vi "Starter Kit 2.0 Robot Receiver.vi"() -> ()   [LabVIEW 2010]
doc: "This VI runs on the Starter Kit RT target. Run this VI before running the host controller VI. You can build this VI into a startup application so that it runs on the robot whenever the RT target is powered on."
uses:
  <vilib>/Platform/TimedLoop/XDataNode/XDataNode.xnode
  <vilib>/Platform/TimedLoop/XDataNode/timing_clust.ctl
  <vilib>/Platform/TimedLoop/XDataNode/nitl_modes.ctl
  <vilib>/Platform/TimedLoop/XDataNode/wakeup.ctl
  Support VIs/Motor Velocity.ctl
  <vilib>/robotics/Starter Kit/2.0/9632 Host Interface/NI_Robotics_Starter Kit Host_9632_2.0.lvclass
  <vilib>/Platform/TimedLoop/XDataNode/XDNodeRunTimeDep.lvlib
  <vilib>/robotics/Starter Kit/Host Interface/NI_Robotics_Starter Kit Host.lvclass
  <vilib>/NI_Real-Time Target Support.lvlib
panel:
  out "connection":i32
  in  "stop":bool
  in  "port (12345)":u16=12345
  in  "ccw servo angle (rad)":dbl
  in  "right motor ccw vel sp":dbl
  in  "left motor ccw vel sp":dbl
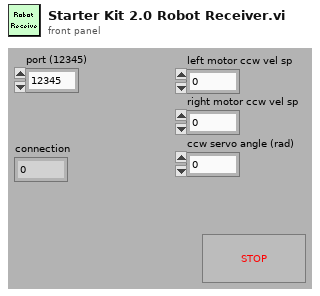
[diagram p1: front panel]
types:
  T1 = typedef "XDNodeRunTimeDep.lvlib/timing_clust.ctl" = cluster{"Expected End [f-1]":u64, "Actual End [f-1]":u64, "Finished Late? [f-1]":bool, "Expected End [i-1]":u64, "Actual End [i-1]":u64, "Finished Late? [i-1]":bool, "Expected Start [i]":u64, "Actual Start [i]":u64, "Expected Start [f]":u64, "Actual Start [f]":u64, "Source Name":string, "Structure Name":string, "Period":i64, "Deadline":i64, "Offset":i64, "Start":i64, "Priority":i32, "Timeout":i32, "Mode":T2, "Wakeup Reason":T3, "Error":errorcluster, "Source Type":string, "Secondary Source Type":string, "Global End Time":u64, "Global Start Time":u64, "Frame Duration":u64, "Iteration Duration":u64, "Assigned CPU":i32, "I/O Scan Engine Mode":u32}
  T2 = typedef "XDNodeRunTimeDep.lvlib/nitl_modes.ctl" = enum32{"No Change", "Process missed periods, maintain original phase", "Discard missed periods, maintain original phase", "Process missed periods, ignore original phase", "Discard missed periods, ignore original phase"}
  T3 = typedef "XDNodeRunTimeDep.lvlib/wakeup.ctl" = enum32{"Normal", "Aborted", "Asynchronous wakeup", "Timing source error", "Timed loop error", "Timeout"}
  T4 = typedef "Motor Velocity.ctl" = cluster{"left motor ccw vel":dbl, "right motor ccw vel":dbl}
  T5 = typedef "Starter Kit Message.ctl" = cluster{"message type":enum16{"Heartbeat", "Motor Vel SP", "Servo Angle", "Stop"}, "message data":variant}
  T6 = enum16{"Heartbeat", "Motor Vel SP", "Servo Angle", "Stop"}
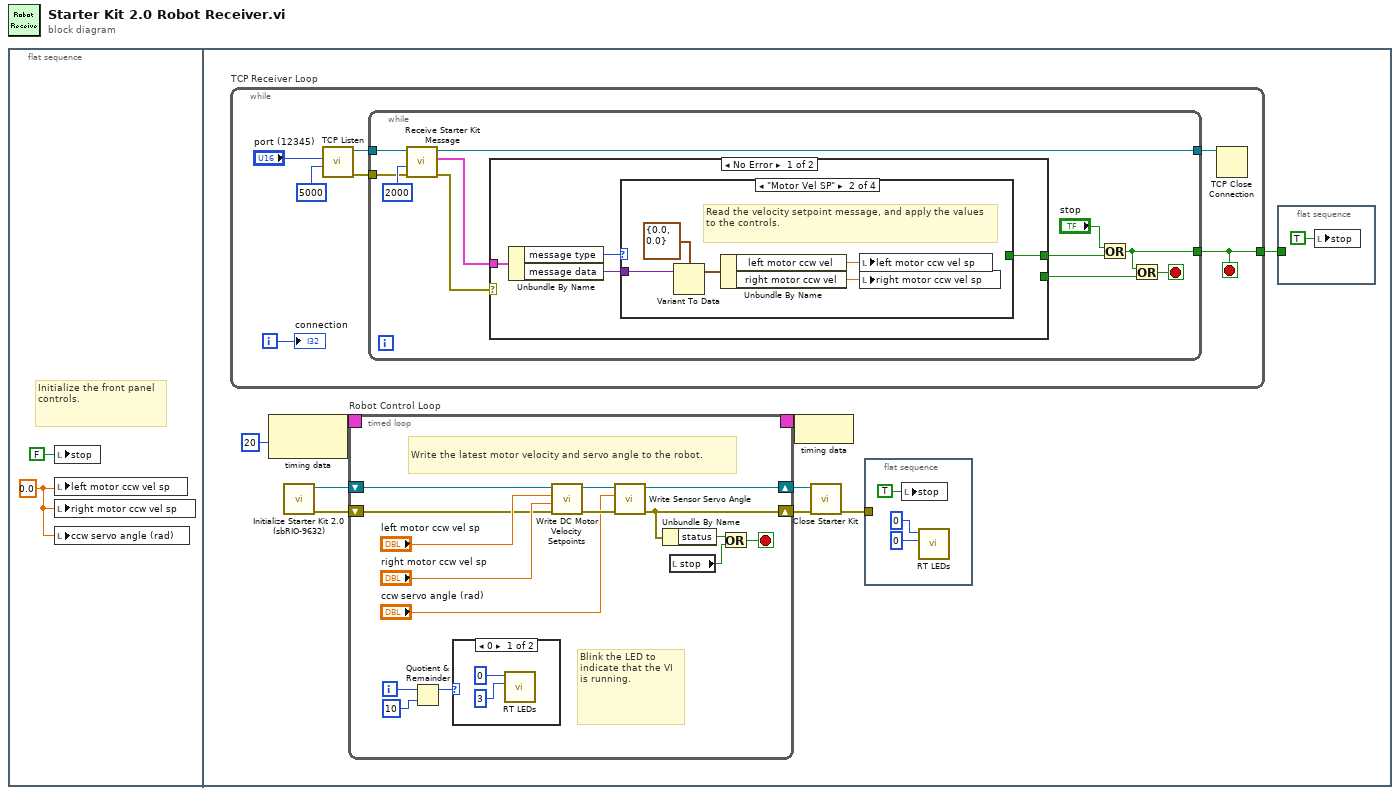
[diagram p0: block diagram]
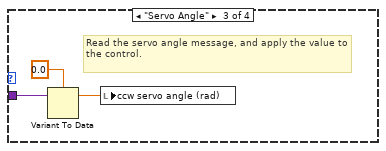
[diagram p4: hidden frame]
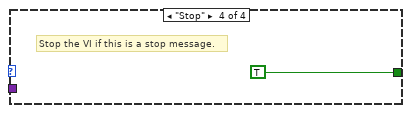
[diagram p5: hidden frame]
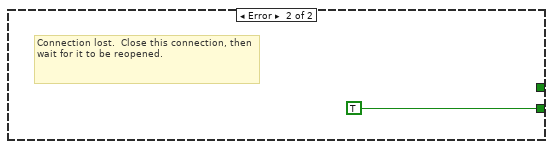
[diagram p6: hidden frame]
diagram:
  n1 = flat-sequence {
    frame #0 {
      w1 = 0.0 ("left motor ccw vel sp")
      # "Initialize the front panel controls."
      n2 = local write "stop"(FALSE ("stop")) -> ()
      n3 = local write "left motor ccw vel sp"(w1) -> ()
      n4 = local write "right motor ccw vel sp"(w1) -> ()
      n5 = local write "ccw servo angle (rad)"(w1) -> ()
    }
    frame #1 {
      n6 = while "TCP Receiver Loop" {
        tunnel: [w40] -> w11
        i -> [w39]
        stop <- w40 stop-if-true
        n7 = call <vilib>:"TCP Listen.vi"("timeout ms (wait forever: -1)"=5000, "port"="port (12345)") -> ("error out"=w41:errorcluster, "connection ID"=w44:refnum<k5>)  [unwired: 2 in, 6 out]
        n8 = while {
          tunnel: w44 -> [w54]
          tunnel: [w53] -> w43
          tunnel: [w48] -> w40
          tunnel: w41 -> [w49]
          stop <- w46 stop-if-true
          n9 = call "Receive Starter Kit Message.vi"("error in (no error)"=w49, "timeout ms (25000)"=2000, "connection ID in"=w54) -> ("error out"=w50:errorcluster, "message"=w52:T5, "connection ID out"=w53:refnum<k5>)  [unwired: 6 in]
          n10 = case shown="No Error" w50 {
            tunnel: [w58 _] -> w55
            tunnel: w52 -> [w57 _]
            tunnel: [_ TRUE] -> w47
            frame No Error {
              n11 = Unbundle By Name(w57) -> ("message type"=w60:T6, "message data"=w59:variant)
              n12 = case shown="\"Motor Vel SP\"" w60 {
                tunnel: w59 -> [_ w65 w67 _]
                tunnel: [_ _ _ TRUE] -> w58
                frame "Heartbeat", Default {
                  # "Do nothing if the message is a heartbeat."
                }
                frame "Motor Vel SP" {
                  # "Read the velocity setpoint message, and apply the values to the controls."
                  n13 = Variant To Data(Variant=w65, type=T4 {"left motor ccw vel"=0.0, "right motor ccw vel"=0.0} ("motor velocity")) -> (data=w63:T4)  [unwired: 1 in, 1 out]
                  n14 = Unbundle By Name(w63) -> ("left motor ccw vel"=w62:dbl, "right motor ccw vel"=w61:dbl)
                  n15 = local write "left motor ccw vel sp"(w62) -> ()
                  n16 = local write "right motor ccw vel sp"(w61) -> ()
                }
                frame "Servo Angle" {
                  # "Read the servo angle message, and apply the value to the control."
                  n17 = Variant To Data(Variant=w67, type=0.0) -> (data=w66:dbl)  [unwired: 1 in, 1 out]
                  n18 = local write "ccw servo angle (rad)"(w66) -> ()
                }
                frame "Stop" {
                  # "Stop the VI if this is a stop message."
                }
              }
            }
            frame Error {
              # "Connection lost.  Close this connection, then wait for it to be reopened."
            }
          }
          n19 = Or(x="stop", y=w55) -> (x .or. y?=w48:bool)
          n20 = Or(x=w48, y=w47) -> (x .or. y?=w46:bool)
        }
        n21 = TCP Close Connection(connection ID=w43) -> ()  [unwired: 1 in, 3 out]
        "connection" <- w39
      }
      n22 = node-c288(i64 20 ("Period")) -> (w10:T1)
      n23 = call <vilib>:"Initialize Starter Kit 2.0 (sbRIO-9632).vi"() -> ("error out"=w3:errorcluster, "FPGA starter kit host 2.0 out"=w4:refnum<class "NI_Robotics_Starter Kit Host_9632_2.0.lvclass">)  [unwired: 10 in]
      n24 = timed-loop "Robot Control Loop" {
        timing: w10 -> [_]
        timing-out: [_] -> w9
        shift-right: [w22] -> w7
        shift-left: w4 -> [w29]
        shift-right: [w21] -> w6
        shift-left: w3 -> [w26]
        i -> [w17]
        stop <- w18 stop-if-true
        # "Write the latest motor velocity and servo angle to the robot."
        # "Blink the LED to indicate that the VI is running."
        n25 = Quotient & Remainder(x=w17, y=10) -> (x-y*floor(x/y)=w15:i32)  [unwired: 1 out]
        n26 = case shown="0" w15 {
          frame 0 {
            n27 = call <vilib>:"RT LEDs.vi"("State"=3, "LED Num"=0) -> ()  [unwired: 4 in, 2 out]
          }
          frame Default {
          }
        }
        n28 = call <vilib>:"Write DC Motor Velocity Setpoints.vi"("error in (no error)"=w26, "right motor ccw velocity (rad/s)"="right motor ccw vel sp", "left motor ccw velocity (rad/s)"="left motor ccw vel sp", "starter kit host in"=w29) -> ("error out"=w24:errorcluster, "starter kit host out"=w25:refnum<class "NI_Robotics_Starter Kit Host_9632_2.0.lvclass">)  [unwired: 6 in]
        n29 = call <vilib>:"Write Sensor Servo Angle.vi"("error in (no error)"=w24, "ccw servo angle (rad)"="ccw servo angle (rad)", "starter kit host in"=w25) -> ("error out"=w21:errorcluster, "starter kit host out"=w22:refnum<class "NI_Robotics_Starter Kit Host_9632_2.0.lvclass">)  [unwired: 7 in]
        n30 = Unbundle By Name(w21) -> ("status"=w20:bool)
        n31 = local read "stop"() -> (w19:bool)
        n32 = Or(x=w20, y=w19) -> (x .or. y?=w18:bool)
      }
      n33 = node-c288(w9) -> ()
      n34 = call-dynamic "Close Starter Kit.vi"("error in (no error)"=w6, "starter kit host in"=w7) -> ("error out"=w5:errorcluster)  [unwired: 9 in]
      n35 = flat-sequence {
        tunnel: w5 -> [_]
        frame #0 {
          n36 = local write "stop"(TRUE ("stop")) -> ()
          n37 = call <vilib>:"RT LEDs.vi"("State"=0, "LED Num"=0) -> ()  [unwired: 4 in, 2 out]
        }
      }
      n38 = flat-sequence {
        tunnel: w11 -> [_]
        frame #0 {
          n39 = local write "stop"(TRUE ("stop")) -> ()
        }
      }
    }
  }
